vi "Delete Table.vi"(8 "error in":errorcluster, 10 "Table Path":string, 11 "LV-Data.PGSQL":refnum<class "LV-Data.PGSQL.lvclass">) -> (0 "error out":errorcluster, 3 "LV-Data.PGSQL out":refnum<class "LV-Data.PGSQL.lvclass">)   [LabVIEW 2019, in "LV-Data.PGSQL.lvclass"]
uses:
  LV-Data.PGSQL.lvclass
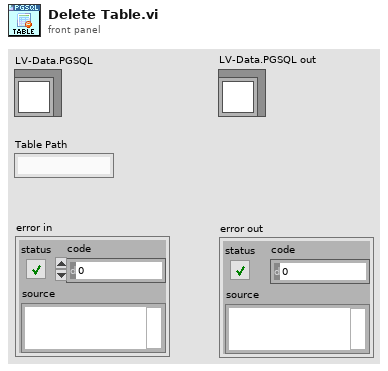
[diagram p1: front panel]
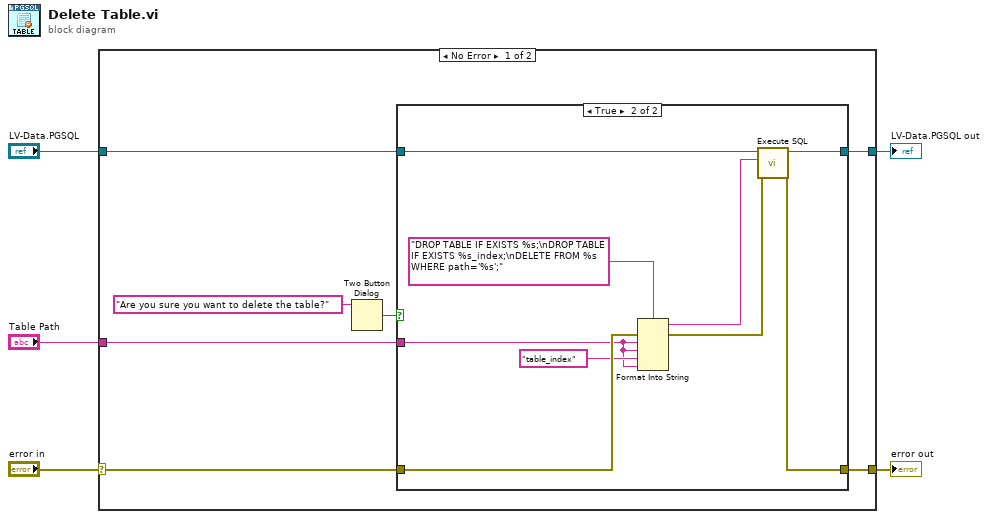
[diagram p0: block diagram]
diagram:
  n1 = case shown="No Error" "error in" {
    selector: "error in" -> [w12 w25]
    tunnel: "LV-Data.PGSQL" -> [w11 w24]
    tunnel: [w10 w25] -> w3
    tunnel: [w9 w24] -> w2
    tunnel: "Table Path" -> [w8 _]
    frame No Error {
      n2 = Two Button Dialog(message="Are you sure you want to delete the table?") -> (T button?=w7:bool)  [unwired: 2 in]
      n3 = case shown="True" w7 {
        tunnel: w12 -> [w13 w20]
        tunnel: w11 -> [w14 w19]
        tunnel: [w13 w18] -> w10
        tunnel: [w14 w17] -> w9
        tunnel: w8 -> [_ w15]
        frame False {
        }
        frame True {
          n4 = Format Into String(format string="DROP TABLE IF EXISTS %s;\nDROP TABLE IF EXISTS %s_index;\nDELETE FROM %s WHERE path='%s';", error in=w20, w15, w15, "table_index" ("input 3"), w15) -> (resulting string=w22:string, error out=w21:errorcluster)  [unwired: 1 in]
          n5 = call "Execute SQL.vi"("error in"=w21, "SQL"=w22, "LV-Data.PGSQL"=w19) -> ("error out"=w18:errorcluster, "LV-Data.PGSQL out"=w17:refnum<class "LV-Data.PGSQL.lvclass">)  [unwired: 5 in, 2 out]
        }
      }
    }
    frame Error {
    }
  }
  "error out" <- w3
  "LV-Data.PGSQL out" <- w2
